vi "Single Z Ramp Retreat Experiment.vi"(0 "Experimental Queue":T1) -> ()   [LabVIEW 2013]
uses:
  Runtime/Runtime Queue.ctl
  Runtime/Experimental Configuration.ctl
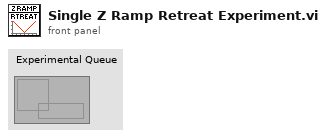
[diagram p1: front panel]
types:
  T1 = typedef "Runtime Queue.ctl" = refnum<queue>
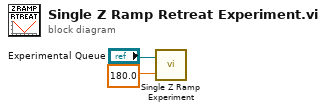
[diagram p0: block diagram]
diagram:
  n1 = call "Single Z Ramp Experiment.vi"("Initial Phase Offset"=180.0 ("Phase Offset"), "Experimental Queue"="Experimental Queue") -> ()
